vi "Build_Mask Write Holding Register.vi"(5 "OR mask":u16, 7 "AND mask":u16, 8 "error in (no error)":errorcluster, 10 "starting address":u16) -> (0 "error out":errorcluster, 3 "MB_PDU":T1={"Function Code"=1, "Data"=[], "RTU_DataBytes"=0})   [LabVIEW 2016, in "MB Master.lvlib"]
doc: "Builds PDU for Mask Write Register (function code 22)."
uses:
  MB Master.lvlib
  MB_PDU_Cluster.ctl
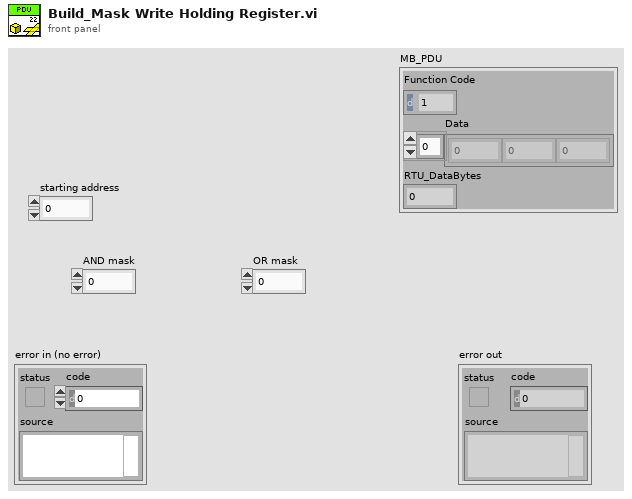
[diagram p1: front panel]
types:
  T1 = typedef "MB Master.lvlib/MB_PDU_Cluster.ctl" = cluster{"Function Code":u8, "Data":u8[], "RTU_DataBytes":i32}
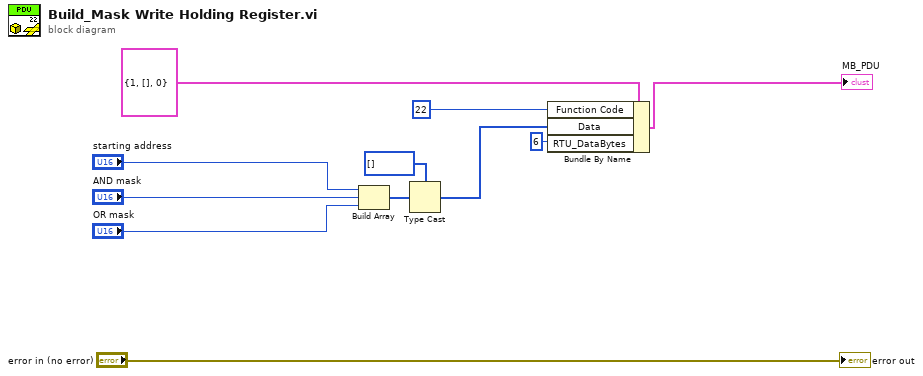
[diagram p0: block diagram]
diagram:
  n1 = Build Array("starting address", "AND mask", "OR mask") -> (w11:u16[])
  n2 = Type Cast(type=u8[] [], x=w11) -> (*(type *) &x=w2:u8[])
  n3 = Bundle By Name(cluster=T1 {"Function Code"=1, "Data"=[], "RTU_DataBytes"=0} ("Modbus Serial New.lvlib:MB_PDU.lvclass"), "Function Code"=u8 22, "Data"=w2, "RTU_DataBytes"=6 ("NumBytes")) -> (→"MB_PDU":T1)
  "error out" <- "error in (no error)"
